vi "Create File.vi"(7 "Run Data":T7={"Target Folder"=path "", "Menu Folder"=path "", "Active Folder"=path "", "Config"={"Main"={"Menu Folder"="", "Re-Create Menu Folder?"=FALSE, "Allow mnu replace?"=FALSE}, "File Filter"={"Exclude Prefixes"=[], "Ignore Names"=[], "Include Extensions"=[], "Exclude Postfixes"=[]}, "Folder Filter"={"Exclude Prefixes"=[], "Ignore Names"=[]}, "File Name Edit"={"Pre Split String"="", "Post Split String"="", "Deletion Strings"=[]}, "Folder Name Edit"={"Pre Split String"="", "Post Split String"="", "Deletion Strings"=[]}, "Folder Icon Map"={}, "Default Palette Data"={"Display Name Override"="", "View Format"=2, "Palette Width"=0, "Help Tag"="", "Help File Path"=path "", "Palette Description"=""}, "Default File Data"={"Display Name Override"="", "Place VI Contents?"=FALSE}, "Palette Override map"={}, "File Override map"={}}} {"Config"."Default Palette Data"."View Format" items=["Icons", "Text", "Icons and Text"]}, 8 "error in (no error)":errorcluster, 11 "palette data":T1 {"view format" items=["Icons", "Text", "Icons and Text"]}) -> (0 "error out":errorcluster, 3 "deleted path":path)   [LabVIEW 2019, in "AutoMenuCreator.lvlib"]
uses:
  AutoMenuCreator.lvlib
  Ctl/Ctl_Run Data.ctl
  Ctl/Ctl_Config.ctl
  Ctl/Ctl_Config_Main.ctl
  Ctl/Ctl_Config_File Filter.ctl
  Ctl/Ctl_Config_Folder Filter.ctl
  Ctl/Ctl_Config_Name Edit.ctl
  Ctl/Ctl_Config_Folder Icon Map.ctl
  Ctl/Ctl_Config_Palette Data.ctl
  <vilib>/Palette API/Palette Menu/Public Type Define/View Format.ctl
  Ctl/Ctl_Config_File Data.ctl
  <vilib>/Palette API/Palette Menu/Public Type Define/Palette Data.ctl
  <vilib>/Palette API/Palette Menu/Public Type Define/Items.ctl
  <vilib>/Palette API/Palette Menu/Public Type Define/Item.ctl
  <vilib>/Palette API/Palette Menu/Public Type Define/Help Info.ctl
  <vilib>/Palette API/Palette Menu/Public Type Define/Synchronize Info.ctl
  <vilib>/Palette API/Palette Menu/Public Type Define/Palette type.ctl
  <vilib>/Palette API/Palette Menu/Palette Menu.lvlib
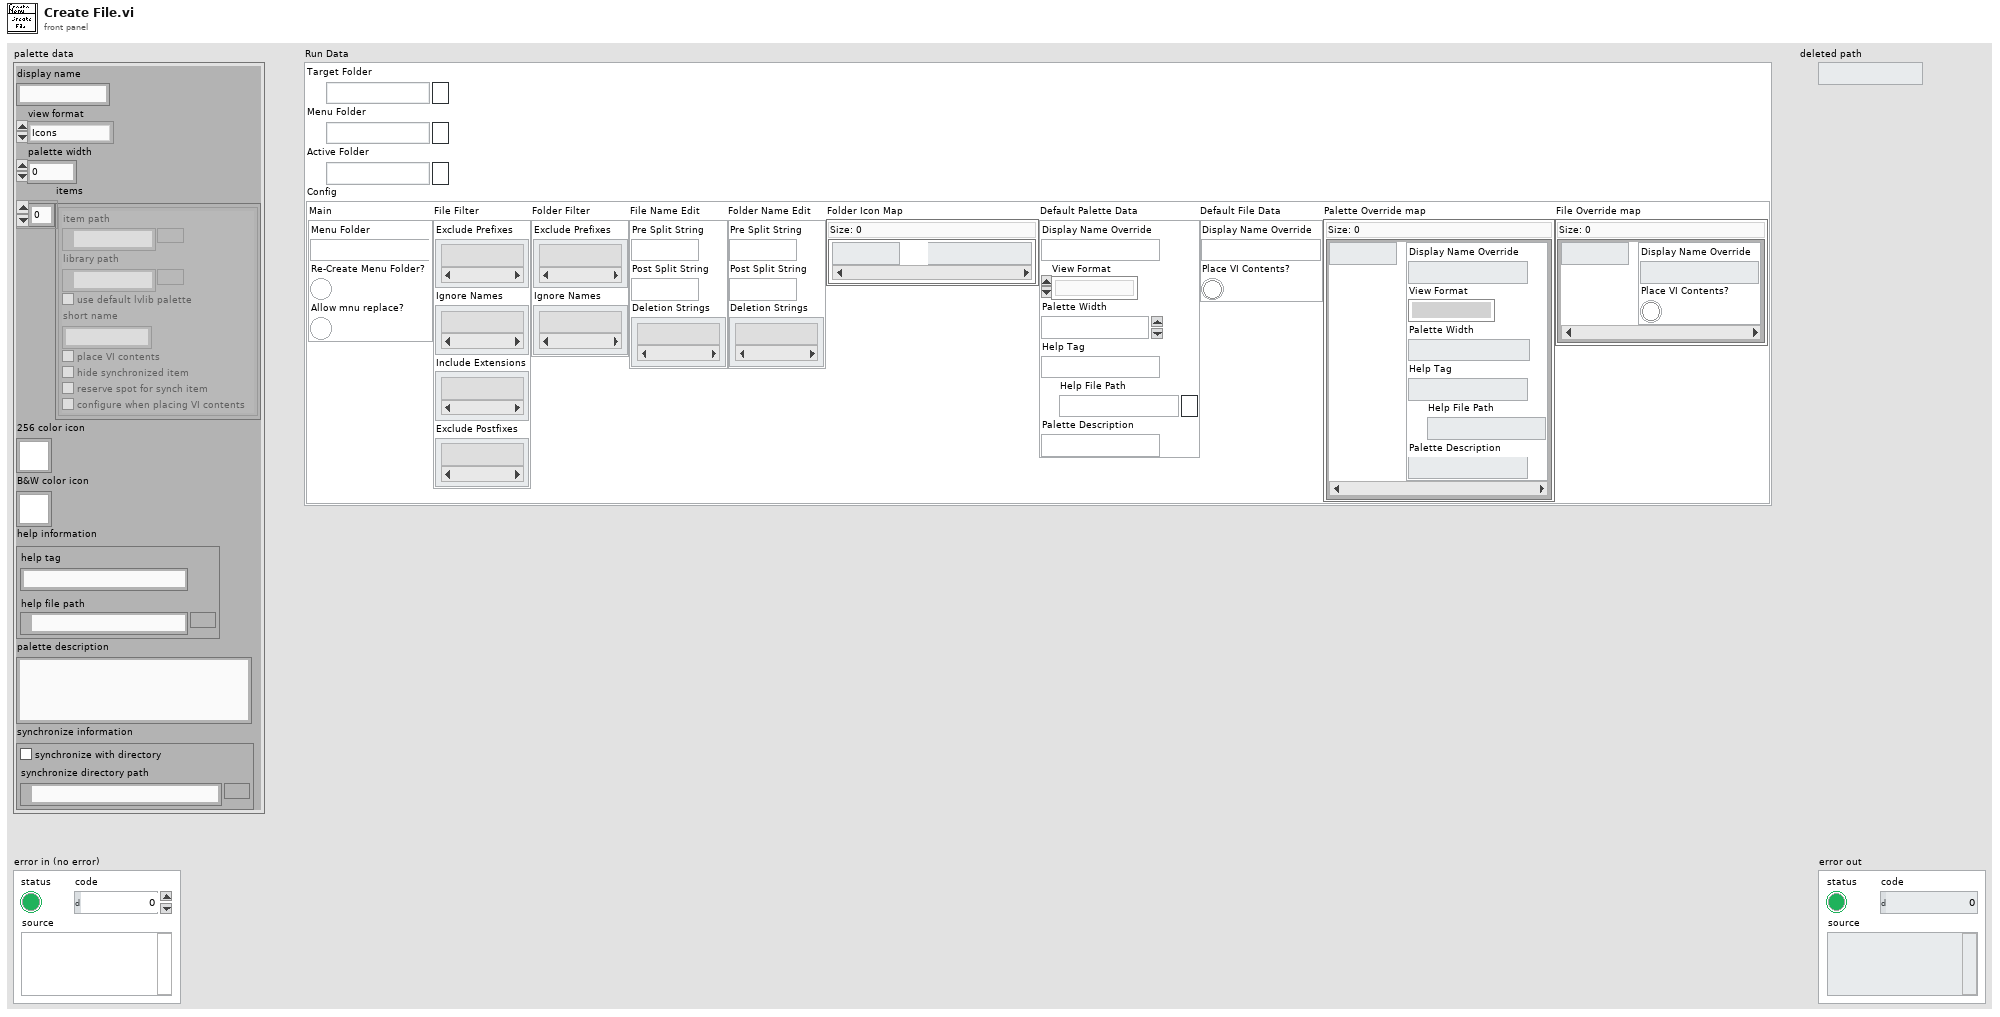
[diagram p1: front panel]
types:
  T1 = typedef "Palette Menu.lvlib/Palette Data.ctl" = cluster{"display name":string, "view format":T2, "palette width":i16, "items":T3, "256 color icon":picture, "B&W color icon":picture, "help information":T5, "palette description":string, "synchronize information":T6}
  T2 = typedef "Palette Menu.lvlib/View Format.ctl" = u16
  T3 = typedef "Palette Menu.lvlib/Items.ctl" = T4[]
  T4 = typedef "Palette Menu.lvlib/Item.ctl" = cluster{"item path":path, "library path":path, "use default lvlib palette":bool, "short name":string, "place VI contents":bool, "hide synchronized item":bool, "reserve spot for synch item":bool, "configure when placing VI contents":bool}
  T5 = typedef "Palette Menu.lvlib/Help Info.ctl" = cluster{"help tag":string, "help file path ":path}
  T6 = typedef "Palette Menu.lvlib/Synchronize Info.ctl" = cluster{"synchronize with directory":bool, "synchronize directory path":path}
  T7 = typedef "AutoMenuCreator.lvlib/Ctl_Run Data.ctl" = cluster{"Target Folder":path, "Menu Folder":path, "Active Folder":path, "Config":T8}
  T8 = typedef "AutoMenuCreator.lvlib/Ctl_Config.ctl" = cluster{"Main":T9, "File Filter":T10, "Folder Filter":T11, "File Name Edit":T12, "Folder Name Edit":T12, "Folder Icon Map":T13, "Default Palette Data":T14, "Default File Data":T15, "Palette Override map":map{string, T14}, "File Override map":map{string, T15}}
  T9 = typedef "AutoMenuCreator.lvlib/Ctl_Config_Main.ctl" = cluster{"Menu Folder":string, "Re-Create Menu Folder?":bool, "Allow mnu replace?":bool}
  T10 = typedef "AutoMenuCreator.lvlib/Ctl_Config_File Filter.ctl" = cluster{"Exclude Prefixes":string[], "Ignore Names":string[], "Include Extensions":string[], "Exclude Postfixes":string[]}
  T11 = typedef "AutoMenuCreator.lvlib/Ctl_Config_Folder Filter.ctl" = cluster{"Exclude Prefixes":string[], "Ignore Names":string[]}
  T12 = typedef "AutoMenuCreator.lvlib/Ctl_Config_Name Edit.ctl" = cluster{"Pre Split String":string, "Post Split String":string, "Deletion Strings":string[]}
  T13 = typedef "AutoMenuCreator.lvlib/Ctl_Config_Folder Icon Map.ctl" = map{string, path}
  T14 = typedef "AutoMenuCreator.lvlib/Ctl_Config_Palette Data.ctl" = cluster{"Display Name Override":string, "View Format":T2, "Palette Width":i16, "Help Tag":string, "Help File Path":path, "Palette Description":string}
  T15 = typedef "AutoMenuCreator.lvlib/Ctl_Config_File Data.ctl" = cluster{"Display Name Override":string, "Place VI Contents?":bool}
  T16 = typedef "Palette Menu.lvlib/Palette type.ctl" = i32
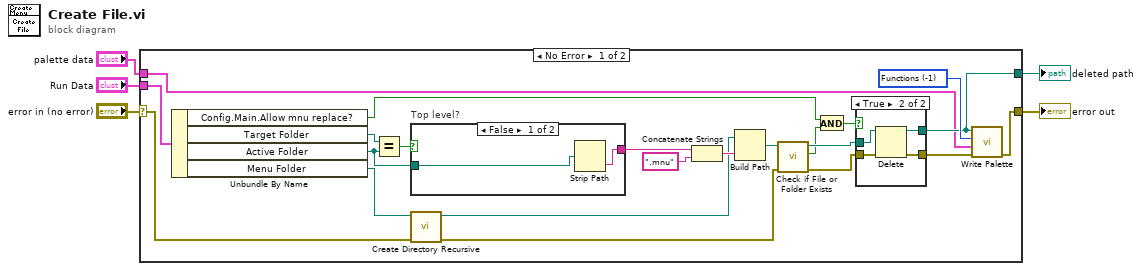
[diagram p0: block diagram]
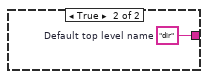
[diagram p2: hidden frame]
diagram:
  n1 = case shown="No Error" "error in (no error)" {
    selector: "error in (no error)" -> [w10 w37]
    tunnel: "Run Data" -> [w22 _]
    tunnel: [w18 _] -> w4
    tunnel: [w7 w37] -> w2
    tunnel: "palette data" -> [w6 _]
    frame No Error {
      w21 = T16 -1 items=["Functions"=-1, "Controls"=-2] ("palette type")
      n2 = Unbundle By Name(w22) -> ("Config.Main.Allow mnu replace?"=w20:bool, "Target Folder"=w23:path, "Active Folder"=w26:path, "Menu Folder"=w27:path)
      n3 = Equal?(x=w23, y=w26) -> (x = y?=w24:bool)
      n4 = case "Top level?" shown="False" w24 {
        tunnel: [w28 w30] -> w25
        tunnel: w26 -> [w29 _]
        frame False {
          n5 = Strip Path(path=w29) -> (name=w28:string)  [unwired: 1 out]
        }
        frame True {
          w30 = "dir"  # Default top level name
        }
      }
      n6 = call <vilib>:"Create Directory Recursive.vi"("error in (no error)"=w10, "directory"=w27) -> ("error out"=w8:errorcluster, "directory copy"=w9:path)  [unwired: 3 in, 1 out]
      n7 = Concatenate Strings(w25, ".mnu" ("file name(dir.mnu)")) -> (w12:string)
      n8 = Build Path(base path=w9, name or relative path=w12) -> (appended path=w13:path)
      n9 = call <vilib>:"Check if File or Folder Exists.vi"("error in (no error)"=w8, "path"=w13) -> ("error out"=w15:errorcluster, "file or folder exists?"=w14:bool, "dup path"=w17:path)  [unwired: 7 in]
      n10 = And(x=w20, y=w14) -> (x .and. y?=w19:bool)
      n11 = case shown="True" w19 {
        tunnel: [w32 w35] -> w16
        tunnel: w15 -> [w32 w36]
        tunnel: w17 -> [w31 w34]
        tunnel: [w31 w33] -> w18
        frame False {
        }
        frame True {
          n12 = Delete(path (use dialog)=w34, error in=w36) -> (deleted path=w33:path, error out=w35:errorcluster)  [unwired: 3 in, 1 out]
        }
      }
      n13 = call <vilib>:"Write Palette.vi"("error in (no error)"=w16, "palette data"=w6, "palette type"=w21, "palette path"=w18) -> ("error out"=w7:errorcluster)  [unwired: 7 in]
    }
    frame Error {
    }
  }
  "deleted path" <- w4
  "error out" <- w2
